vi "LK-G5000 GetCalcData.vi"() -> ()   [LabVIEW 8.6]
uses:
  Keyence LK-G5000.lvlib
  Public/Constant/Comm Interface.ctl
  Public/enum/LKIF_OUTNO.ctl
  Public/enum/LKIF_FLOATRESULT.ctl
panel:
  out "Trend Graph":cluster{"[0]":sgl, "[1]":sgl, "[2]":sgl}(graph)
  in  "Stop VI":bool
  out "CalcData":T2(array[cluster]) {"LKIF_FLOATRESULT" items=["VALID", "RANGEOVER_P", "RANGEOVER_N", "WAITING", "ALARM", "INVALID"]}
  in  "OutNo 3":T3 items=["OUT01", "OUT02", "OUT03", "OUT04", "OUT05", "OUT06", "OUT07", "OUT08", "OUT09", "OUT10", "OUT11", "OUT12", "ALL OUT"]
  in  "OutNo 2":T3 items=["OUT01", "OUT02", "OUT03", "OUT04", "OUT05", "OUT06", "OUT07", "OUT08", "OUT09", "OUT10", "OUT11", "OUT12", "ALL OUT"]
  in  "OutNo":T3 items=["OUT01", "OUT02", "OUT03", "OUT04", "OUT05", "OUT06", "OUT07", "OUT08", "OUT09", "OUT10", "OUT11", "OUT12", "ALL OUT"]
  in  "IP Address":u8[](array[numeric])
  in  "Comm Interface":T4
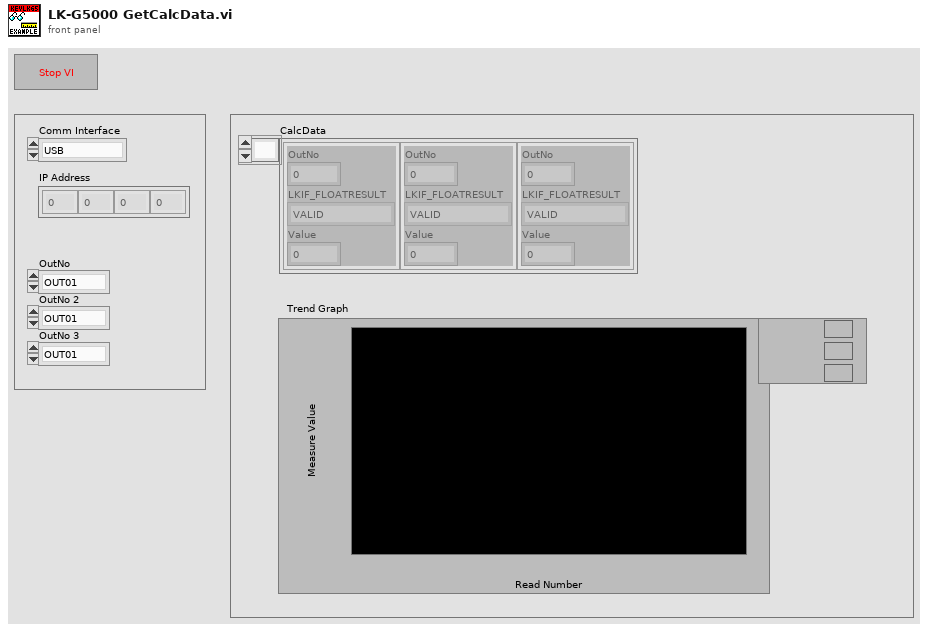
[diagram p1: front panel]
types:
  T1 = typedef "Keyence LK-G5000.lvlib/LKIF_FLOATRESULT.ctl" = i32
  T2 = cluster{"OutNo":i32, "LKIF_FLOATRESULT":T1, "Value":sgl}[]
  T3 = typedef "Keyence LK-G5000.lvlib/LKIF_OUTNO.ctl" = i32
  T4 = typedef "Keyence LK-G5000.lvlib/Comm Interface.ctl" = enum8{"USB", "ETHERNET"}
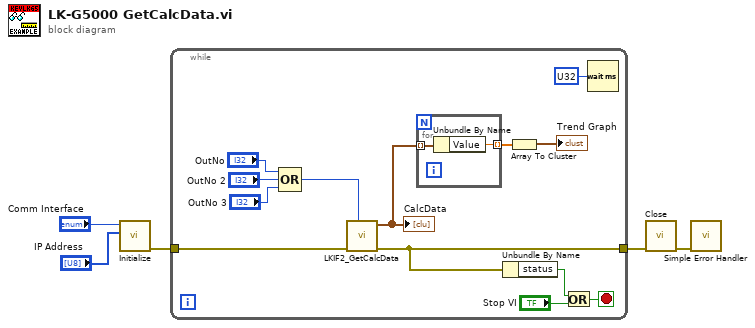
[diagram p0: block diagram]
diagram:
  n1 = call "Initialize.vi"("IP Address"="IP Address", "Comm Interface"="Comm Interface") -> ("error out"=w5:errorcluster)  [unwired: 9 in]
  n2 = while {
    tunnel: w5 -> [w18]
    tunnel: [w16] -> w4
    stop <- w17 stop-if-true
    n3 = Compound Arithmetic op=OR("OutNo", "OutNo 2", "OutNo 3") -> (w10:T3)
    n4 = call "LKIF2_GetCalcData.vi"("OutNo (OUT1)"=w10, "error in (no error)"=w18) -> ("error out"=w16:errorcluster, "CalcData"=w9:T2)  [unwired: 8 in]
    "CalcData" <- w9
    n5 = for {
      tunnel: w9 -> [w20] mode=indexing
      tunnel: [w19] -> w8 mode=indexing
      n6 = Unbundle By Name(w20) -> ("Value"=w19:sgl)
    }
    n7 = Unbundle By Name(w16) -> ("status"=w15:bool)
    n8 = Array To Cluster(array=w8) -> (cluster=→"Trend Graph":cluster{"[0]":sgl, "[1]":sgl, "[2]":sgl})
    n9 = Or(x=w15, y="Stop VI") -> (x .or. y?=w17:bool)
    n10 = Wait (ms)(milliseconds to wait=u32 ? ("ミリ秒待機時間")) -> ()  [unwired: 1 out]
  }
  n11 = call "Close.vi"("error in (no error)"=w4) -> ("error out"=w1:errorcluster)  [unwired: 10 in]
  n12 = call <vilib>:"Simple Error Handler.vi"("error in (no error)"=w1) -> ()  [unwired: 4 in, 5 out]
